vi "SerialStepForce.vi"() -> ()   [LabVIEW 2017]
uses:
  <vilib>/Utility/file.llb/Read Delimited Spreadsheet (string).vi
  <vilib>/Utility/file.llb/Write Delimited Spreadsheet (string).vi
panel:
  out "Change Port":bool
  out "RX Serial Bytes":u32
  out "NEW RX":bool caption="RX OK"
  in  "BAUDRATE":string(combo)="19200"
  in  "COMPORT":string(combo)="COM4"
  out "PortOK":bool
  out "StepForce":u8[](array[numeric])
  out "RX OK":bool
  in  "Refresh":bool
  in  "Exit":bool
  out "TimeNew RX":i32
  # "Door Lock/Unlock 1"
  # "FR Up/Down 1"
  # "RR Up/Down 1"
  # "FL Up/Down 1"
  # "RL Up/Down 1"
  # "Door Lock/Unlock 2"
  # "FR Up/Down 2"
  # "RR Up/Down 2"
  # "FL Up/Down 2"
  # "RL Up/Down 2"
  # "WDW Lock/Unlock 1"
  # "WDW Lock/Unlock 2"
  # "STEP FORCE"
  # "STEP FORCE"
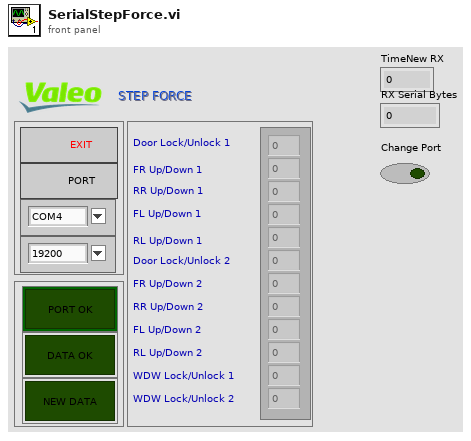
[diagram p1: front panel]
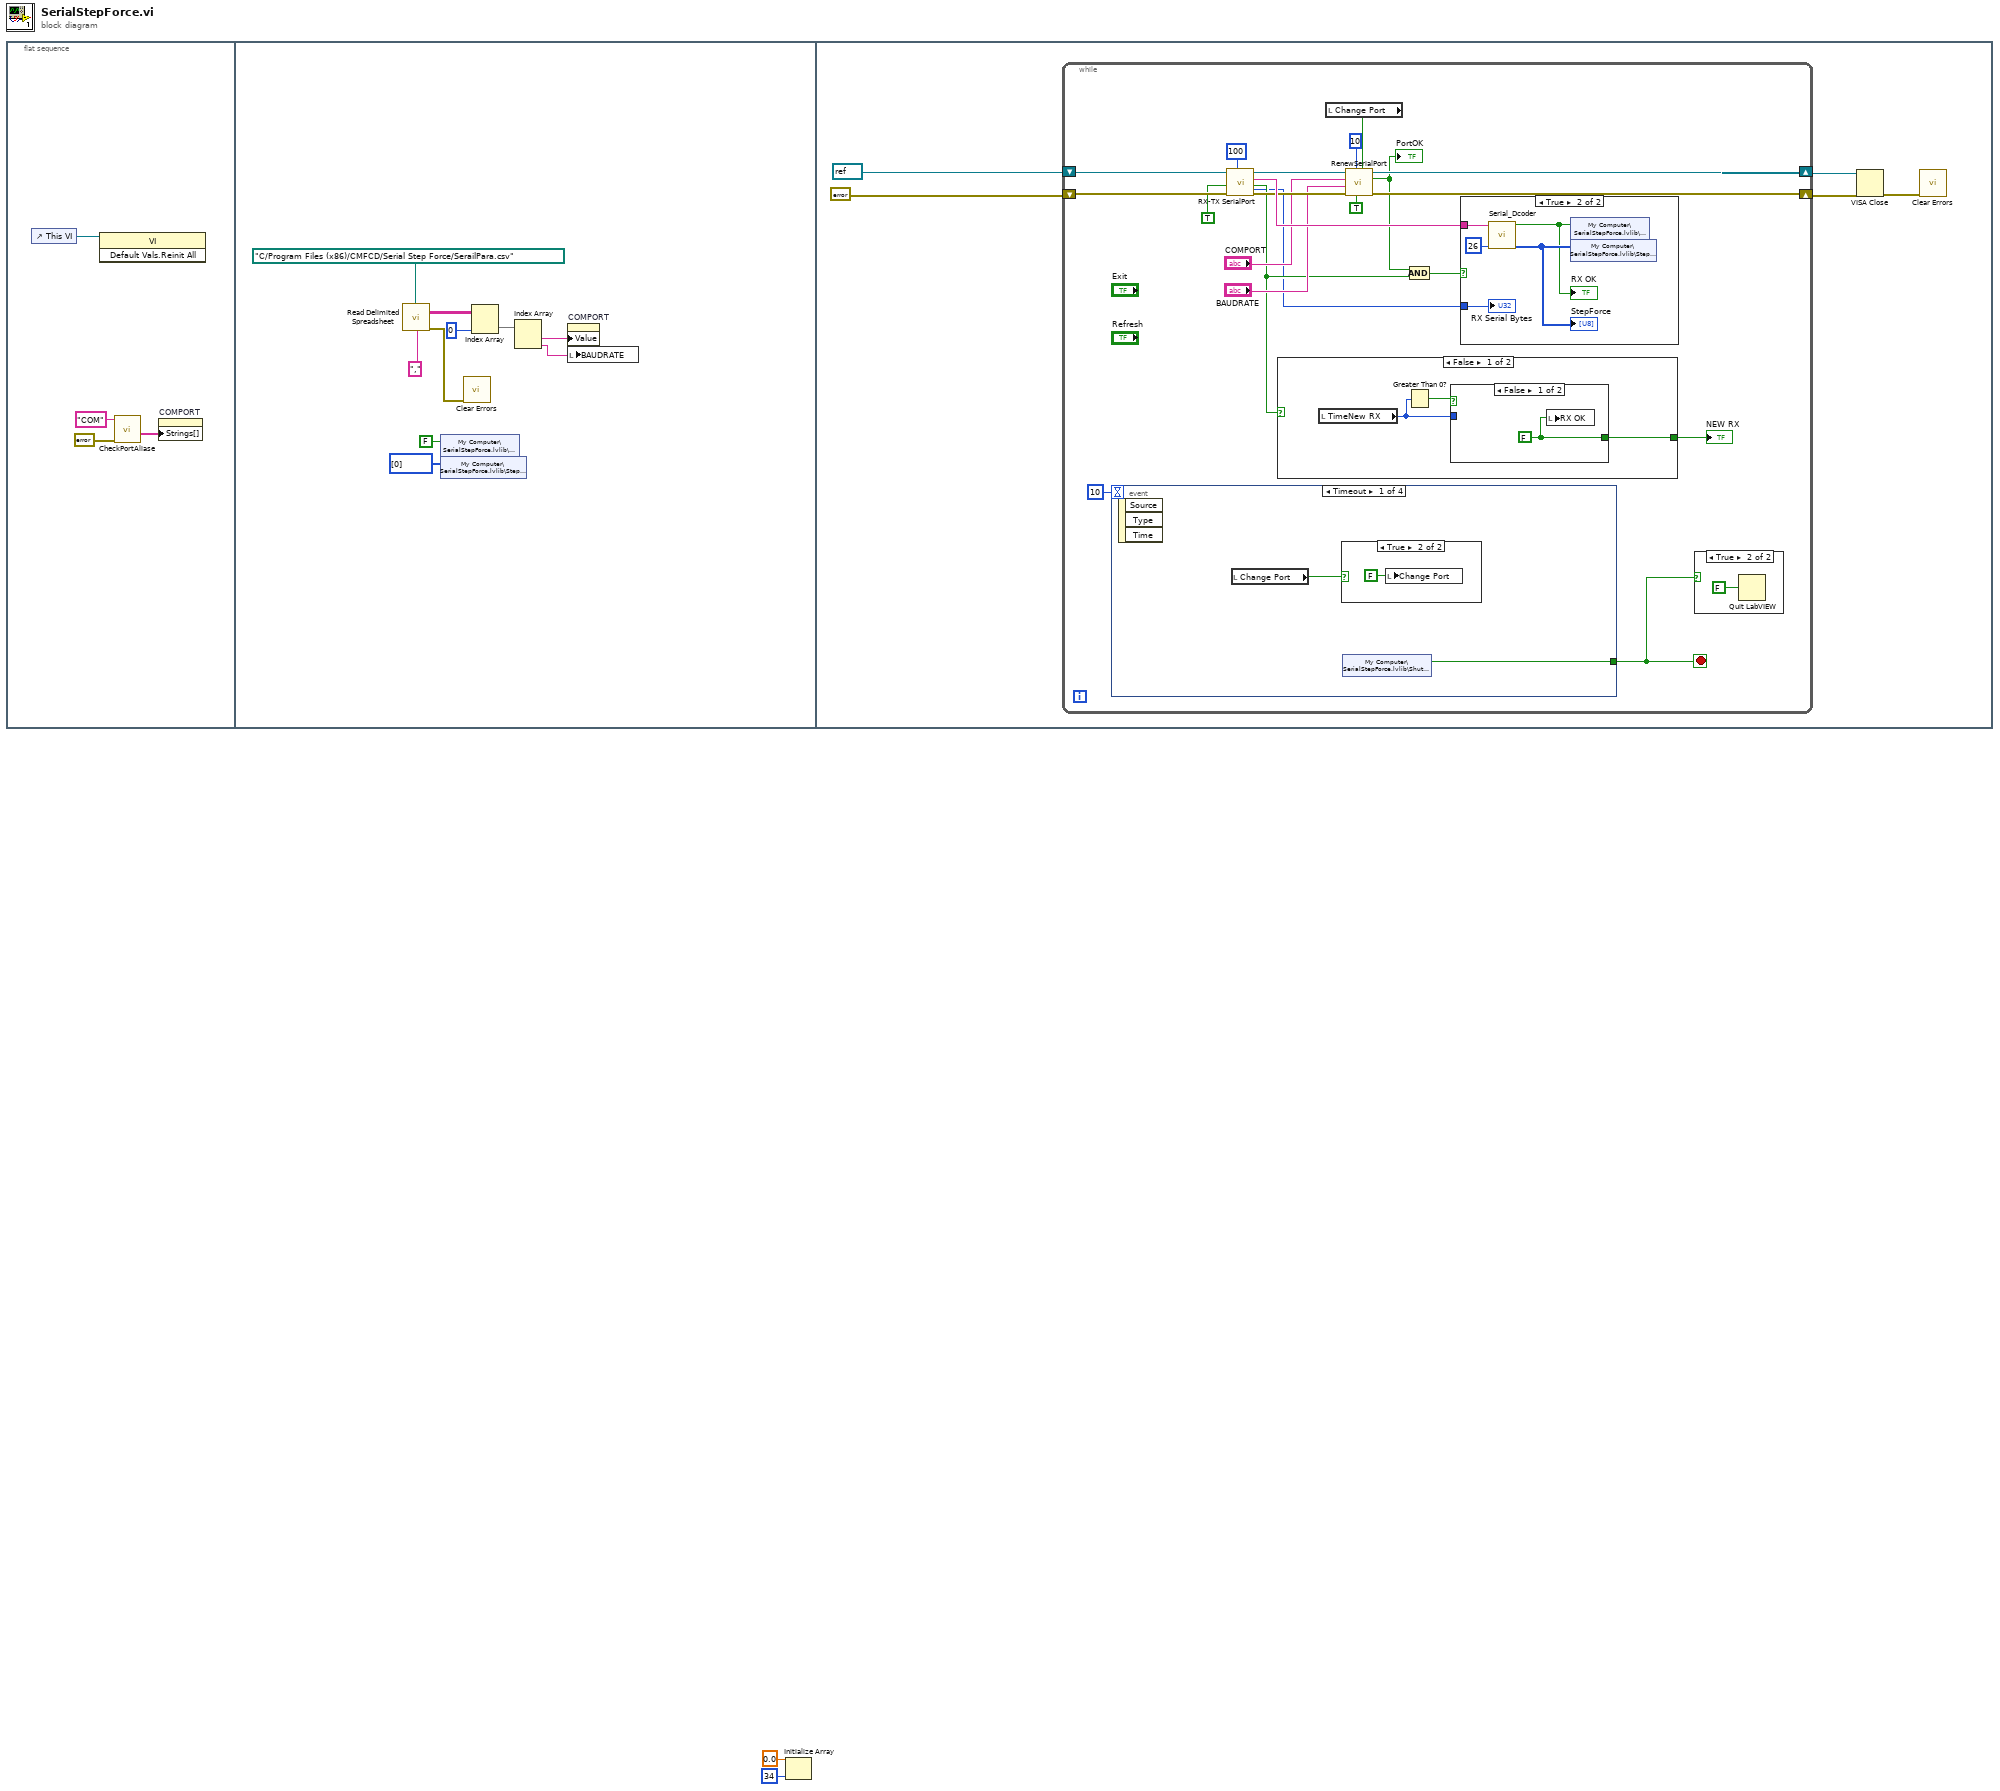
[diagram p0: block diagram]
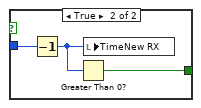
[diagram p2: hidden frame]
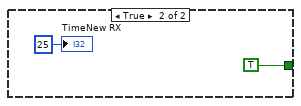
[diagram p3: hidden frame]
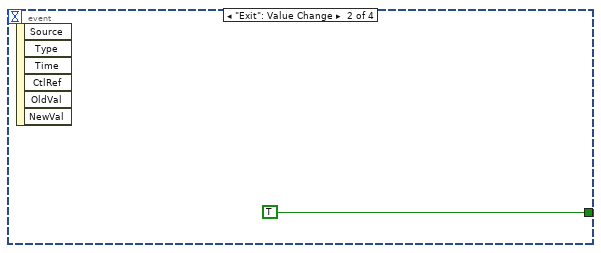
[diagram p7: hidden frame]
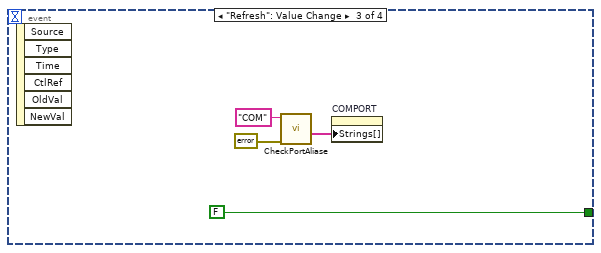
[diagram p8: hidden frame]
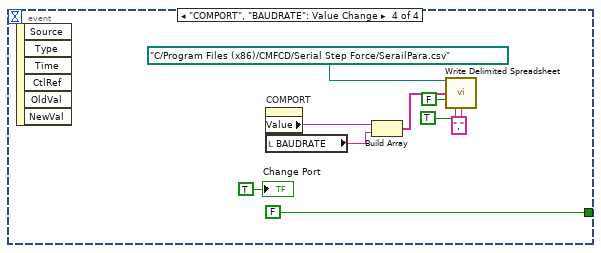
[diagram p9: hidden frame]
diagram:
  n1 = flat-sequence {
    frame #0 {
      n2 = control-ref of="This VI"() -> (w6:refnum<vi>)
      n3 = invoke class="VI" method="Default Vals.Reinit All"(reference=w6) -> ()  [unwired: 2 in, 3 out]
      n4 = call "CheckPortAliase.vi"("error in"=errorcluster {"status"=FALSE, "code"=0, "source"=""}, "ComPortName"="COM") -> ("Port list"=w3:string[])  [unwired: 4 in, 5 out]
      n5 = property on="COMPORT" class="CmbBox"("Strings[]"=w3) -> ()  [unwired: 2 in, 2 out]
    }
    frame #1 {
      n6 = call-poly <vilib>:"Read Delimited Spreadsheet.vi"("file path (dialog if empty)"=path "C:/Program Files (x86)/CMFCD/Serial Step Force/SerailPara.csv", "delimiter (\\t)"="," ("delimiter (\\t)")) -> ("all rows"=w15:string[][], "error out"=w16:errorcluster)  [unwired: 8 in, 4 out]
      n7 = shared-variable "My Computer\\SerialStepForce.lvlib\\Serial OK"(FALSE ("Serial OK")) -> ()  [unwired: 1 in, 1 out]
      n8 = shared-variable "My Computer\\SerialStepForce.lvlib\\Step Force"(u8[] [0] ("Step Force")) -> ()  [unwired: 1 in, 1 out]
      n9 = call <vilib>:"Clear Errors.vi"("error in (no error)"=w16) -> ()  [unwired: 5 in, 2 out]
      n10 = Index Array(array=w15, index (col)=0 ("disabled index (col)")) -> (element=w7:string[])  [unwired: 1 in]
      n11 = Index Array(array=w7) -> (element #1=w8:string, element #2=w9:string)  [unwired: 2 in]
      n12 = property on="COMPORT" class="CmbBox"("Value"=w8) -> ()  [unwired: 2 in, 2 out]
      n13 = local write "BAUDRATE"(w9) -> ()
    }
    frame #2 {
      n14 = while {
        shift-right: [w41] -> w21
        shift-left: refnum<visa-resource-name> refnum ("VISA Out") -> [w40]
        shift-right: [w32] -> w20
        shift-left: errorcluster {"status"=FALSE, "code"=0, "source"=""} ("error out") -> [w39]
        stop <- w29 stop-if-true
        n15 = event shown="[0] Timeout" {
          selector: _ -> [_ _ _ _]
          dyn-events: _ -> [_ _ _ _]
          timeout: 10 -> [_ _ _ _]
          tunnel: [w59 TRUE FALSE FALSE] -> w29
          event Timeout {
            n16 = event-data() -> ()  [unwired: 1 in, 3 out]
            n17 = local read "Change Port"() -> (w58:bool)
            n18 = case shown="True" w58 {
              frame False {
              }
              frame True {
                n19 = local write "Change Port"(FALSE ("Change Port")) -> ()
              }
            }
            n20 = shared-variable "My Computer\\SerialStepForce.lvlib\\Shut down"() -> (w59:bool)  [unwired: 1 in, 1 out]
          }
          event "Exit": Value Change {
            n21 = event-data() -> ()  [unwired: 1 in, 6 out]
          }
          event "Refresh": Value Change {
            n22 = event-data() -> ()  [unwired: 1 in, 6 out]
            n23 = call "CheckPortAliase.vi"("error in"=errorcluster {"status"=FALSE, "code"=0, "source"=""}, "ComPortName"="COM") -> ("Port list"=w65:string[])  [unwired: 4 in, 5 out]
            n24 = property on="COMPORT" class="CmbBox"("Strings[]"=w65) -> ()  [unwired: 2 in, 2 out]
          }
          event "COMPORT", "BAUDRATE": Value Change {
            n25 = event-data() -> ()  [unwired: 1 in, 6 out]
            n26 = property on="COMPORT" class="CmbBox"() -> ("Value"=w70:string)  [unwired: 2 in, 2 out]
            n27 = local read "BAUDRATE"() -> (w74:string)
            n28 = Build Array(w70, w74) -> (w73:string[])
            n29 = call-poly <vilib>:"Write Delimited Spreadsheet.vi"("file path (dialog if empty)"=path "C:/Program Files (x86)/CMFCD/Serial Step Force/SerailPara.csv", "1D data"=w73, "append to file? (new file:F)"=FALSE, "transpose? (no:F)"=TRUE, "delimiter (\\t)"="," ("delimiter (\\t)")) -> ()  [unwired: 9 in, 2 out]
            "Change Port" <- TRUE ("Change Port")
          }
        }
        n30 = call "RX-TX SerialPort.vi"("Byte RX"=u32 100, "Error In"=w39, "Enable"=TRUE, "VISA In"=w40) -> ("Error out"=w35:errorcluster, "NewRX"=w26:bool, "RX Data"=w37:string, "VISA Out"=w36:refnum<visa-resource-name>, "RX Serial Bytes"=w24:u32)  [unwired: 2 in, 1 out]
        n31 = case shown="False" w26 {
          tunnel: [w45 TRUE] -> w25
          frame False {
            n32 = local read "TimeNew RX"() -> (w43:i32)
            n33 = Greater Than 0?(x=w43) -> (x > 0?=w44:bool)
            n34 = case shown="False" w44 {
              tunnel: [w46 w48] -> w45
              tunnel: w43 -> [_ w47]
              frame False {
                w46 = FALSE
                n35 = local write "RX OK"(w46) -> ()
              }
              frame True {
                n36 = Decrement(x=w47) -> (x-1=w49:i32)
                n37 = Greater Than 0?(x=w49) -> (x > 0?=w48:bool)
                n38 = local write "TimeNew RX"(w49) -> ()
              }
            }
          }
          frame True {
            "TimeNew RX" <- 25 ("TimeNew RX")
          }
        }
        "NEW RX" <- w25
        n39 = local read "Change Port"() -> (w22:bool)
        n40 = call "RenewSerialPort.vi"("Immediate"=w22, "Enable Termination\nChar (T)"=TRUE ("Enable Termination\nChar (T)"), "termination char\n(0xA = '\\n' = LF)"=u8 10 ("termination char\n(0xA = '\\n' = LF)"), "Error in"=w35, "BaudRate"="BAUDRATE", "COMPort"="COMPORT", "VISA In"=w36) -> ("error out"=w32:errorcluster, "PortOK"=w27:bool, "VISA Out"=w41:refnum<visa-resource-name>)  [unwired: 2 in]
        "PortOK" <- w27
        n41 = And(x=w27, y=w26) -> (x .and. y?=w28:bool)
        n42 = case shown="True" w28 {
          tunnel: w37 -> [_ w54]
          tunnel: w24 -> [_ w52]
          frame False {
          }
          frame True {
            n43 = call "Serial_Dcoder.vi"("RX Count"=u32 26, "string"=w54) -> ("StepForce"=w56:u8[], "OK"=w55:bool)  [unwired: 8 in]
            "RX OK" <- w55
            "StepForce" <- w56
            n44 = shared-variable "My Computer\\SerialStepForce.lvlib\\Serial OK"(w55) -> ()  [unwired: 1 in, 1 out]
            n45 = shared-variable "My Computer\\SerialStepForce.lvlib\\Step Force"(w56) -> ()  [unwired: 1 in, 1 out]
            "RX Serial Bytes" <- w52
          }
        }
        n46 = case shown="True" w29 {
          frame False {
          }
          frame True {
            n47 = Quit LabVIEW(quit? (T)=FALSE) -> ()
          }
        }
      }
      n48 = VISA Close(VISA resource name=w21, error in (no error)=w20) -> (error out=w17:errorcluster)
      n49 = call <vilib>:"Clear Errors.vi"("error in (no error)"=w17) -> ()  [unwired: 5 in, 2 out]
    }
  }
  n50 = Initialize Array(0.0 ("element"), 34 ("dimension size")) -> ()  [unwired: 1 out]
